vi "getImage.vi"(0 "hCamera IN":u32, 2 "errorCamera IN":errorcluster, 3 "Image IN":T1, 5 "imageError IN":errorcluster, 8 "Streeam":bool, 9 "Show":bool) -> (14 "hCamera OUT":u32, 15 "1D Data BGR Array OUT":u8[](array[numeric]), 16 "errorCamera OUT":errorcluster, 17 "Image OUT":T1, 18 "1D RGB32 Array OUT":u32[](array[numeric]), 19 "errorImage OUT":errorcluster)   [LabVIEW 2010]
uses:
  <vilib>/vision/Image Controls.llb/IMAQ Image.ctl
  <vilib>/vision/NI_Vision_Development_Module.lvlib
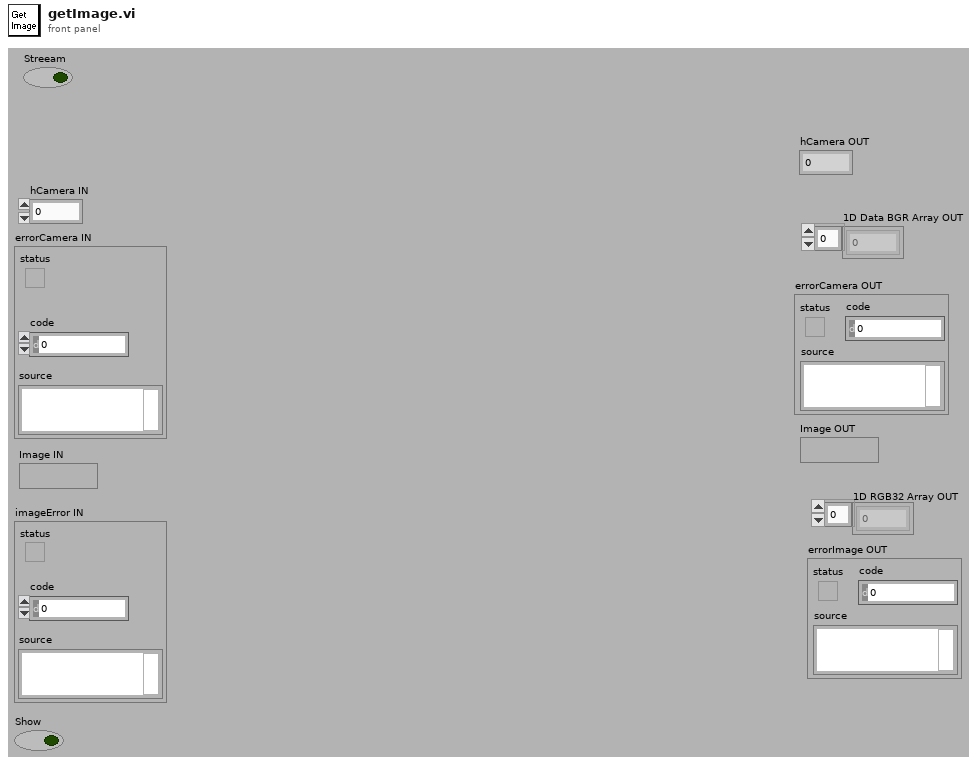
[diagram p1: front panel]
types:
  T1 = typedef "IMAQ Image.ctl" = refnum<image>
  T2 = cluster{"Red or Hue value":u8, "Green or Sat value":u8, "Blue or Luma or Val or Inten value":u8}
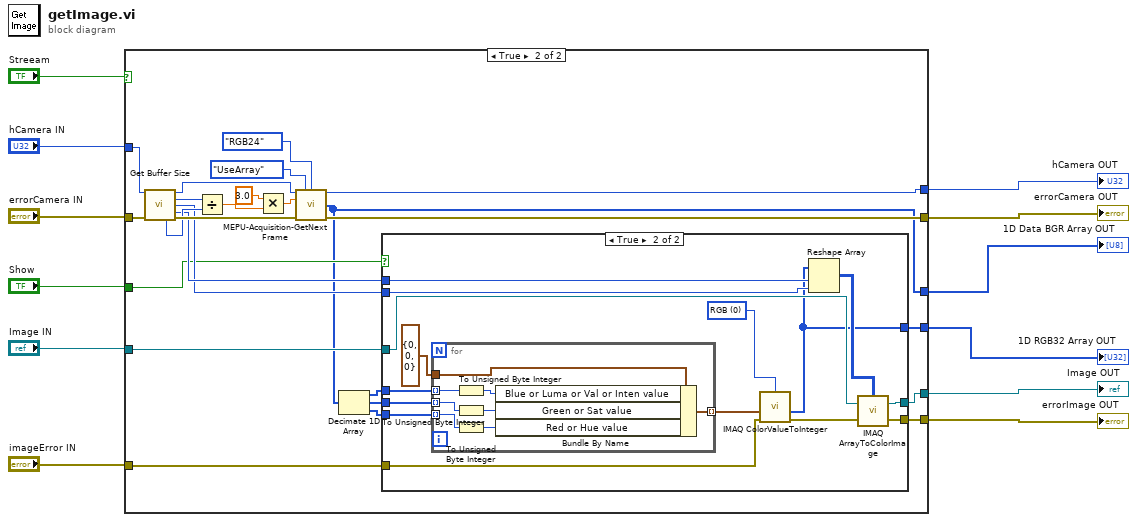
[diagram p0: block diagram]
diagram:
  n1 = case shown="True" "Streeam" {
    tunnel: "hCamera IN" -> [w16 w38]
    tunnel: [w15 w37] -> w7
    tunnel: [w16 w29] -> w4
    tunnel: "errorCamera IN" -> [w15 w36]
    tunnel: "Image IN" -> [w13 w26]
    tunnel: "imageError IN" -> [w14 w23]
    tunnel: [w14 w27] -> w10
    tunnel: [w13 w28] -> w11
    tunnel: "Show" -> [_ w22]
    tunnel: [_ w18] -> w2
    tunnel: [_ w17] -> w1
    frame False {
    }
    frame True {
      n2 = call "Get Buffer Size.vi"("phCamera IN"=w38, "Error IN"=w36) -> ("phCamera OUT"=w39:u32, "uBufferSize OUT"=w31:u32, "uWidth OUT"=w24:u32, "uHeight OUT"=w25:u32, "uBytesPerPixel OUT"=w30:u32, "Error OUT"=w41:errorcluster)  [unwired: 8 out]
      n3 = Divide(x=w31, y=w30) -> (x/y=w33:dbl)
      n4 = Multiply(x=3.0, y=w33) -> (x*y=w34:dbl)
      n5 = call <vilib>:"MEPU-Acquisition-GetNextFrame.vi"("hCamera IN"=w39, "Mode IN"=enum16{"UseArray", "UsePointer"}."UseArray", "OutputMode IN"=enum16{"Default", "RGB24", "RGB32"}."RGB24", "uBufferSize IN"=w34, "Error IN"=w41) -> ("hCamera OUT"=w29:u32, "Data OUT"=w18:u8[], "Error OUT"=w37:errorcluster)  [unwired: 6 in, 2 out]
      n6 = Decimate 1D Array(w18) -> (w21:u8[], w20:u8[], w19:u8[])
      n7 = case shown="True" w22 {
        tunnel: [w42 w48] -> w28
        tunnel: [w43 w58] -> w27
        tunnel: w26 -> [w42 w57]
        tunnel: w25 -> [_ w53]
        tunnel: w24 -> [_ w52]
        tunnel: w23 -> [w43 w49]
        tunnel: w21 -> [_ w47]
        tunnel: w20 -> [_ w46]
        tunnel: w19 -> [_ w45]
        tunnel: [_ w44] -> w17
        frame False {
        }
        frame True {
          w54 = u16 0 items=["RGB", "HSL", "HSV", "HSI"] ("Color Mode")
          n8 = for {
            tunnel: w45 -> [w59] mode=indexing
            tunnel: [w66] -> w55 mode=indexing
            tunnel: T2 {"Red or Hue value"=0, "Green or Sat value"=0, "Blue or Luma or Val or Inten value"=0} ("Color Value") -> [w65]
            tunnel: w47 -> [w60] mode=indexing
            tunnel: w46 -> [w61] mode=indexing
            n9 = To Unsigned Byte Integer(number=w60) -> (unsigned 8bit integer=w62:u8)
            n10 = To Unsigned Byte Integer(number=w61) -> (unsigned 8bit integer=w63:u8)
            n11 = To Unsigned Byte Integer(number=w59) -> (unsigned 8bit integer=w64:u8)
            n12 = Bundle By Name(cluster=w65, "Blue or Luma or Val or Inten value"=w62, "Green or Sat value"=w63, "Red or Hue value"=w64) -> (w66:T2)
          }
          n13 = call "IMAQ ColorValueToInteger"("error in (no error)"=w49, "1D Color value array"=w55, "Color Mode"=w54) -> ("1D U32 array"=w44:u32[], "error out"=w50:errorcluster)  [unwired: 2 in, 2 out]
          n14 = Reshape Array(w44, w53, w52) -> (w51:u32[][])
          n15 = call "IMAQ ArrayToColorImage"("Image Pixels (U32)"=w51, "Image"=w57, "error in (no error)"=w50) -> ("Image Out"=w48:T1, "error out"=w58:errorcluster)  [unwired: 2 in]
        }
      }
    }
  }
  "Image OUT" <- w11
  "errorImage OUT" <- w10
  "errorCamera OUT" <- w7
  "hCamera OUT" <- w4
  "1D Data BGR Array OUT" <- w2
  "1D RGB32 Array OUT" <- w1
